vi "AVS_GetNumPixels.vi"(0 "a_hDevice":i32, 11 "a_pNumPixels":u16) -> (4 "Output Value":i32, 15 "a_pNumPixels":u16)   [LabVIEW 2020]
uses:
  AvaSpecX64-DLL_9.4/avaspecx64.dll
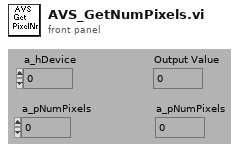
[diagram p1: front panel]
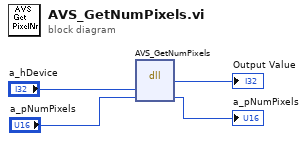
[diagram p0: block diagram]
diagram:
  n1 = dll-call lib="C:/AvaSpecX64-DLL_9.4/avaspecx64.dll" fn="AVS_GetNumPixels"("a_hDevice"="a_hDevice", "a_pNumPixels"="a_pNumPixels") -> ("return type"=→"Output Value":i32, "a_pNumPixels"=→"a_pNumPixels":u16)  [unwired: 4 in, 2 out]
